vi "4.2.1.vi"() -> ()   [LabVIEW 2017]
panel:
  in  "stop":bool
  out "XY Graph":cluster{"X":dbl[], "Y":dbl[]}[](graph)
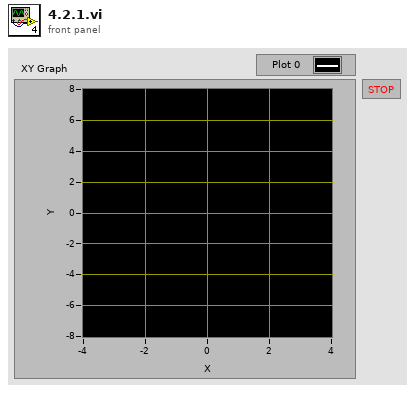
[diagram p1: front panel]
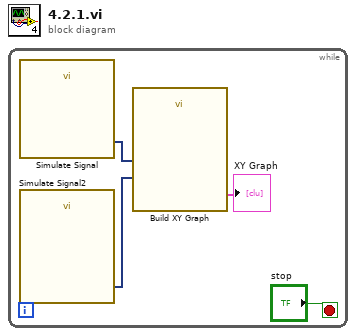
[diagram p0: block diagram]
diagram:
  n1 = while {
    stop <- "stop" stop-if-true
    n2 = call "Simulate Signal"() -> ("Sine"=w4:dynamicdata)  [unwired: 14 in, 1 out]
    n3 = call "Simulate Signal2"() -> ("Sine"=w3:dynamicdata)  [unwired: 14 in, 1 out]
    n4 = call "Build XY Graph"("Y Input"=w3, "X Input"=w4) -> ("XY Graph"=→"XY Graph":cluster{"X":dbl[], "Y":dbl[]}[])  [unwired: 8 in, 1 out]
  }
